vi "读取已用区域引用.vi"(8 "错误输入（无错误）":errorcluster, 10 "表单索引":variant, 11 "所有表单引用":refnum<k7>) -> (0 "错误输出":errorcluster, 1 "选中引用输出":refnum<k7>, 2 "当前表单引用输出":refnum<k7>, 3 "所有表单引用输出":refnum<k7>)   [LabVIEW 2013, in "excel处理.lvlib"]
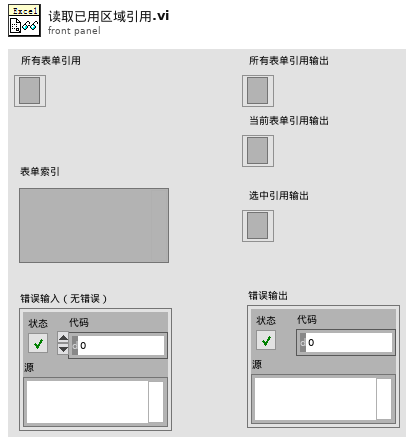
[diagram p1: front panel]
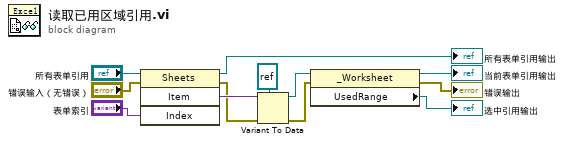
[diagram p0: block diagram]
diagram:
  n1 = invoke on="调用节点" class="Sheets" method="Item"(reference="所有表单引用", error in="错误输入（无错误）", "Index"="表单索引") -> (reference out=→"所有表单引用输出":refnum<k7>, error out=w5:errorcluster, "Item"=w11:variant)  [unwired: 1 in, 1 out]
  n2 = Variant To Data(error in=w5, type=refnum<k7> refnum ("Excel._Worksheet"), Variant=w11) -> (data=w10:refnum<k7>, error out=w4:errorcluster)
  n3 = property on="属性节点" class="_Worksheet"(reference=w10, error in=w4) -> (reference out=→"当前表单引用输出":refnum<k7>, error out=→"错误输出":errorcluster, "UsedRange"=→"选中引用输出":refnum<k7>)
